vi "create.include_id.vi"(10 "IDs":i32[](array[numeric])) -> (3 "Include Filter":refnum<class "include.lvclass">)   [LabVIEW 2020, in "nominal types.lvlib" / "channelFilter.lvlib" / "channelFilter.lvclass"]
uses:
  channelFilter.lvclass
  channelFilter.lvclass/channelFilter.ctl
  include/include.lvclass
  id/id.lvclass
  C:/code/labview-client/lv_src/nominal types/filterTypes/filterTypes.lvclass
  C:/code/labview-client/lv_src/Nominal Client/datasources/payload/payload.lvclass
  C:/code/labview-client/lv_src/nominal types/id/id.lvclass
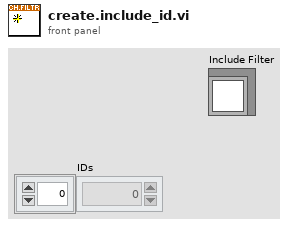
[diagram p1: front panel]
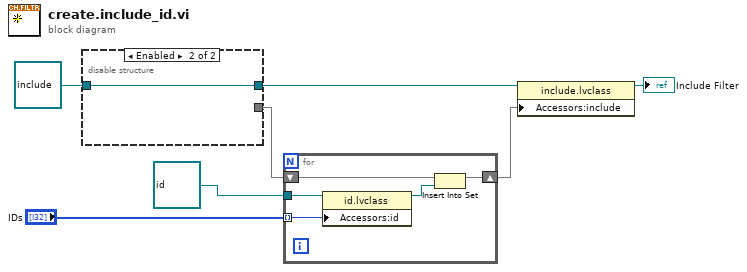
[diagram p0: block diagram]
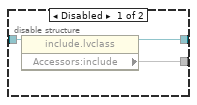
[diagram p2: hidden frame]
diagram:
  n1 = disable-structure shown="Enabled" {
    disable-tunnel: refnum<class "include.lvclass"> refnum ("nominal types.lvlib:channelFilter.lvlib:include.lvclass") -> [w10 w11]
    disable-tunnel: [w9 w11] -> w2
    disable-tunnel: [w8 _] -> w1
    frame Disabled {
      n2 = property class="include.lvclass"(reference=w10) -> (reference out=w9:refnum<class "include.lvclass">, "Accessors:include"=w8:set{refnum<class "filterTypes.lvclass">})  [unwired: 1 in, 1 out]
    }
    frame Enabled {
    }
  }
  n3 = for {
    tunnel: "IDs" -> [w16] mode=indexing
    tunnel: refnum<class "id.lvclass"> refnum ("reference") -> [w15]
    shift-right: [w12] -> w4
    shift-left: w1 -> [w14]
    n4 = property class="id.lvclass"(reference=w15, "Accessors:id"=w16) -> (reference out=w13:refnum<class "id.lvclass">)  [unwired: 1 in, 1 out]
    n5 = Insert Into Set(10:w13, 11:w14) -> (3:w12:set{refnum<class "filterTypes.lvclass">})  [unwired: 1 out]
  }
  n6 = property class="include.lvclass"(reference=w2, "Accessors:include"=w4) -> (reference out=→"Include Filter":refnum<class "include.lvclass">)  [unwired: 1 in, 1 out]
